vi "Get Data.vi"(8 "error in (no error)":errorcluster, 11 "Composite Tree Data in":refnum<class "Composite Tree Data.lvclass">) -> (0 "error out":errorcluster, 3 "Composite Tree Data out":refnum<class "Composite Tree Data.lvclass">)   [LabVIEW 2024, in "Composite Tree Data.lvclass"]
uses:
  Composite Tree Data.lvclass
  Composite Tree Data.lvclass/Composite Tree Data.ctl
  Tree Data/Tree Data.lvclass
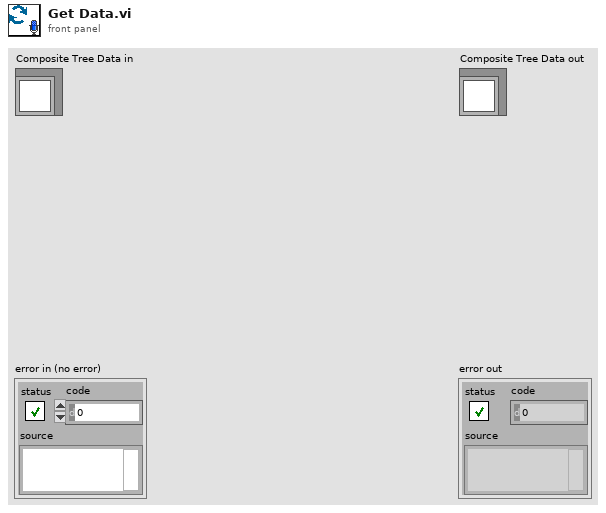
[diagram p1: front panel]
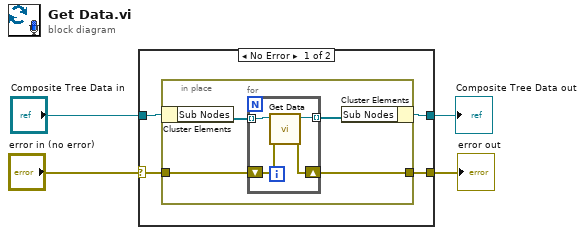
[diagram p0: block diagram]
diagram:
  n1 = case shown="No Error" "error in (no error)" {
    selector: "error in (no error)" -> [w6 w18]
    tunnel: "Composite Tree Data in" -> [w8 w17]
    tunnel: [w5 w18] -> w2
    tunnel: [w7 w17] -> w1
    frame No Error {
      n2 = in-place {
        in-place-border: w6 -> [w10]
        in-place-border: [w9] -> w5
        n3 = in-place-cluster #1(w8) -> ("Sub Nodes"=w12:refnum<class "Tree Data.lvclass">[])
        n4 = for {
          tunnel: w12 -> [w16] mode=indexing
          tunnel: [w15] -> w11 mode=indexing
          shift-right: [w13] -> w9
          shift-left: w10 -> [w14]
          n5 = call-dynamic "Get Data.vi"("error in (no error)"=w14, "Tree Data in"=w16) -> ("error out"=w13:errorcluster, "Tree Data out"=w15:refnum<class "Tree Data.lvclass">)  [unwired: 8 in]
        }
        n6 = in-place-cluster #1("Sub Nodes"=w11) -> (w7:refnum<class "Composite Tree Data.lvclass">)
      }
    }
    frame Error {
    }
  }
  "error out" <- w2
  "Composite Tree Data out" <- w1
